vi "SubModule Acq Stop.vi"(8 "error in (no error)":errorcluster, 11 "Nikon in":refnum<class "Nikon.lvclass">) -> (0 "error out":errorcluster, 3 "Nikon out":refnum<class "Nikon.lvclass">)   [LabVIEW 2021, in "Nikon.lvclass"]
uses:
  Nikon.lvclass
  Camera/Camera.lvclass
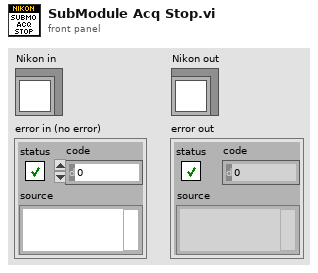
[diagram p1: front panel]
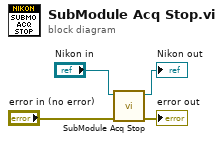
[diagram p0: block diagram]
diagram:
  n1 = call-parent "SubModule Acq Stop.vi"("error in (no error)"="error in (no error)", "Camera in"="Nikon in") -> ("error out"=→"error out":errorcluster, "Camera out"=→"Nikon out":refnum<class "Nikon.lvclass">)  [unwired: 8 in]
